vi "Timestamp to String.vi"(7 "Include Date? (T)":bool=TRUE, 10 "Precision (0)":u8, 11 "time stamp":timestamp) -> (3 "date/time string":string)   [LabVIEW 2018, in "Tag Watchlist.lvlib"]
doc: "_SubVI_"
uses:
  Tag Watchlist.lvlib
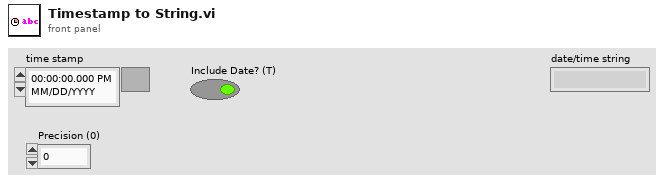
[diagram p1: front panel]
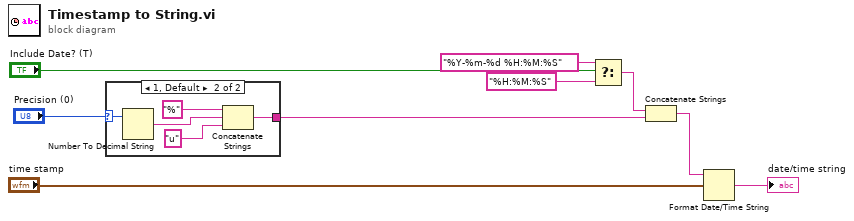
[diagram p0: block diagram]
diagram:
  n1 = case shown="1, Default" "Precision (0)" {
    selector: "Precision (0)" -> [_ w11]
    tunnel: [_ w10] -> w9
    frame 0 {
    }
    frame 1, Default {
      n2 = Number To Decimal String(number=w11) -> (decimal integer string=w13:string)  [unwired: 1 in]
      n3 = Concatenate Strings("%", w13, "u" ("string")) -> (w10:string)
    }
  }
  n4 = Select(t="%Y-%m-%d %H:%M:%S" ("time format string (%c)"), s="Include Date? (T)", f="%H:%M:%S" ("time format string (%c)")) -> (s? t:f=w6:string)
  n5 = Concatenate Strings(w6, w9) -> (w5:string)
  n6 = Format Date/Time String(time format string (%c)=w5, seconds (now)="time stamp") -> (date/time string=→"date/time string":string)  [unwired: 1 in]
